vi "GetTriggerMode.vi"(6 "Delay between send and receive [ms]":i32=100, 8 "error in (no error)":errorcluster, 11 "SCD in":refnum<class "SCD.lvclass">) -> (0 "error out":errorcluster, 2 "TriggerMode":T1, 3 "SCD out":refnum<class "SCD.lvclass">)   [LabVIEW 2023, in "horiba.lvlib" / "SCD.lvclass"]
doc: "Gets the integration time that was previously set. If no integration time has been explicitly set, the default value is returned.\nThe integration time is returned in seconds."
uses:
  SCD.lvclass
  b6349250-cb33-415b-847a-a7f5d99734f6.vi
  a3575502-22b1-481e-8bb0-96f3cfd6d110.vi
  <vilib>/JDP Science/JSONtext/Variant to JSON Text.vi
  <vilib>/JDP Science/JSONtext/Set Item.vi
  <vilib>/JDP Science/JSONtext/JSON text to Variant.vi
  <vilib>/JDP Science/JSONtext/LVClass Serializer/JSONtext LVClass Serializer.lvclass
  GenericDevice/GenericDevice.lvclass
panel:
  # "Connector Pane"
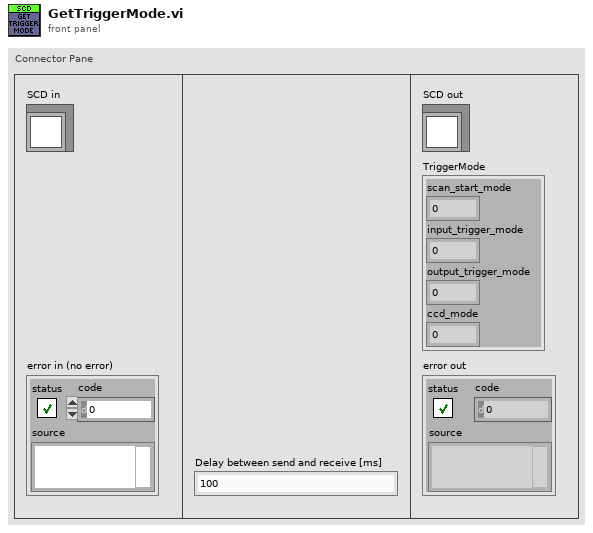
[diagram p1: front panel]
types:
  T1 = cluster{"scan_start_mode":i32, "input_trigger_mode":i32, "output_trigger_mode":i32, "ccd_mode":i32}
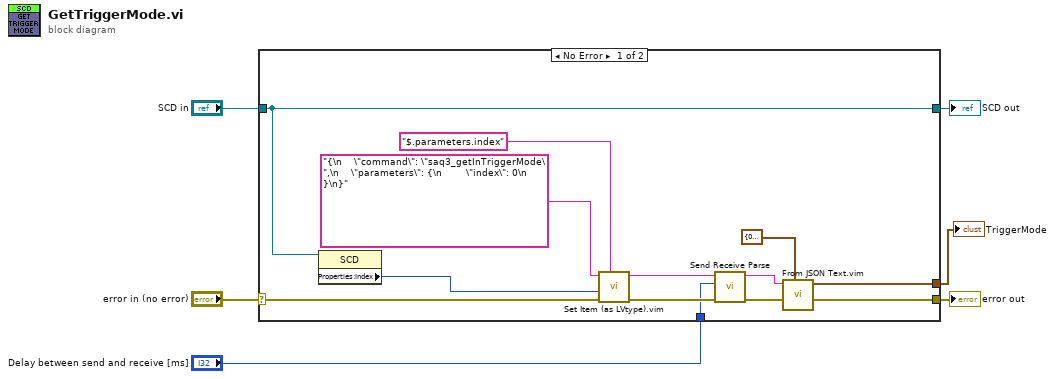
[diagram p0: block diagram]
diagram:
  n1 = case shown="No Error" "error in (no error)" {
    selector: "error in (no error)" -> [w15 w21]
    tunnel: [w14 w21] -> w2
    tunnel: [w17 w20] -> w4
    tunnel: "SCD in" -> [w17 w20]
    tunnel: "Delay between send and receive [ms]" -> [w10 _]
    tunnel: [w7 _] -> w1
    frame No Error {
      n2 = property class="SCD"(reference=w17) -> ("Properties:Index"=w16:i32)  [unwired: 1 in, 2 out]
      n3 = call "Set Item (as LVtype).vim"("$Path or Item Name"="$.parameters.index", "error in (no error)"=w15, "Anything"=w16, "JSON"="{\n    \"command\": \"saq3_getInTriggerMode\",\n    \"parameters\": {\n        \"index\": 0\n    }\n}") -> ("error out"=w12:errorcluster, "<JSON>"=w9:string)  [unwired: 4 in, 1 out]
      n4 = call "Send Receive Parse.vi"("error in"=w12, "Delay between send and receive [ms]"=w10, "<JSON>"=w9) -> ("error out"=w11:errorcluster, "results-JSON string"=w13:string)  [unwired: 6 in, 1 out]
      n5 = call "From JSON Text.vim"("Data Type and Default Value"=T1 {"scan_start_mode"=0, "input_trigger_mode"=0, "output_trigger_mode"=0, "ccd_mode"=0}, "error in (no error)"=w11, "JSON"=w13) -> ("error out"=w14:errorcluster, "Data out"=w7:T1)  [unwired: 7 in]
    }
    frame Error {
    }
  }
  "error out" <- w2
  "SCD out" <- w4
  "TriggerMode" <- w1
